vi "CUST Get PDC Config.vi"(10 "pdcCfg":T1, 11 "pseudoPdcId":i32) -> (2 "pdcCfg out":T1, 3 "function return":i32)   [LabVIEW 2017, in "C37118-DLL.lvlib"]
doc: "STRONGRIDIEEEC37118DLL_API int __cdecl disconnectPdc( int32_t pseudoPdcId);"
uses:
  C37118-DLL.lvlib
  builds/StrongridDLL/StrongridDLL.dll
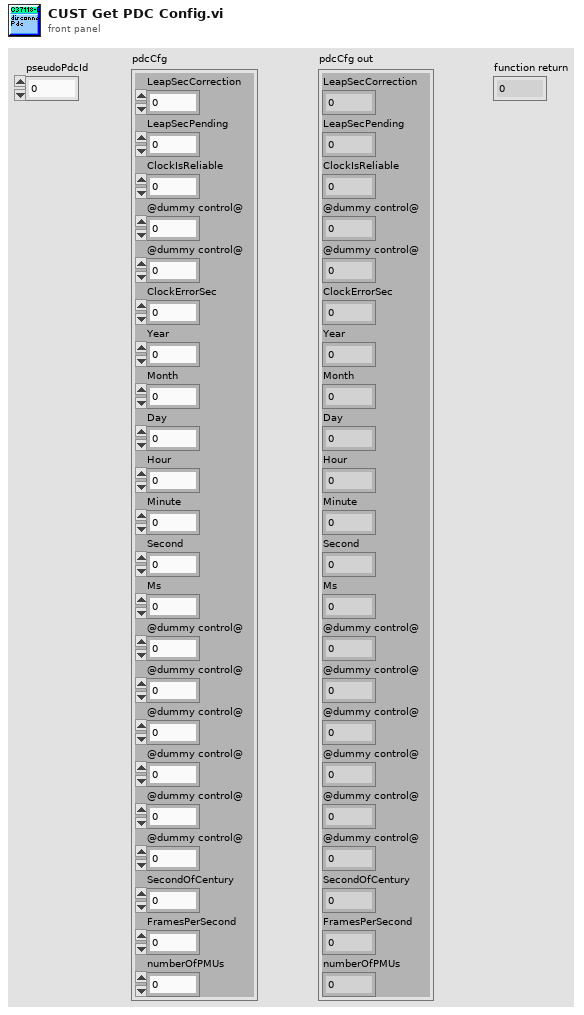
[diagram p1: front panel]
types:
  T1 = cluster{"LeapSecCorrection":i32, "LeapSecPending":u8, "ClockIsReliable":u8, "@dummy control@":i8, "@dummy control@":i8, "ClockErrorSec":sgl, "Year":i16, "Month":i16, "Day":i16, "Hour":i16, "Minute":i16, "Second":i16, "Ms":i16, "@dummy control@":i8, "@dummy control@":i8, "@dummy control@":i8, "@dummy control@":i8, "@dummy control@":i8, "@dummy control@":i8, "SecondOfCentury":dbl, "FramesPerSecond":sgl, "numberOfPMUs":i32}
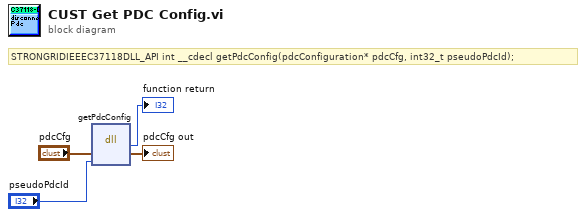
[diagram p0: block diagram]
diagram:
  # "STRONGRIDIEEEC37118DLL_API int __cdecl getPdcConfig(pdcConfiguration* pdcCfg, int32_t pseudoPdcId);"
  n1 = dll-call lib="C:/dev/OSS/S3DK/builds/StrongridDLL/StrongridDLL.*" fn="getPdcConfig"("pdcCfg"="pdcCfg", "pseudoPdcId"="pseudoPdcId") -> (→"function return":i32, "pdcCfg"=→"pdcCfg out":T1)  [unwired: 4 in, 2 out]
